vi "test2.vi"() -> ()   [LabVIEW 2022 SP3]
panel:
  in  "stop":bool
  in  "a":dbl
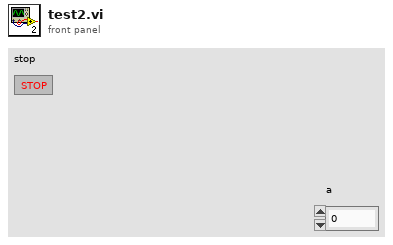
[diagram p1: front panel]
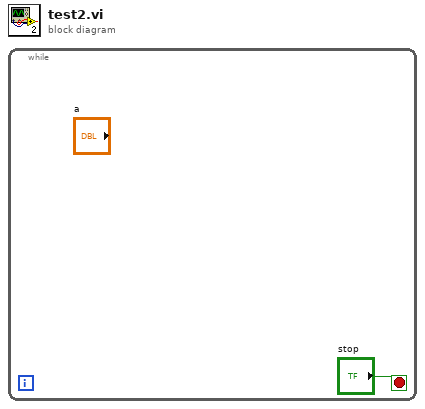
[diagram p0: block diagram]
diagram:
  n1 = while {
    stop <- "stop" stop-if-true
  }
